vi "test2.vi"   [LabVIEW 2012]
uses:
  <vilib>/NXT/Dual Mode Library/Waits/Wait_Num.vi
types:
  T1 = typedef "LVHSConnector.ctl" = cluster{"Hardware":string, "Flattened String":string}
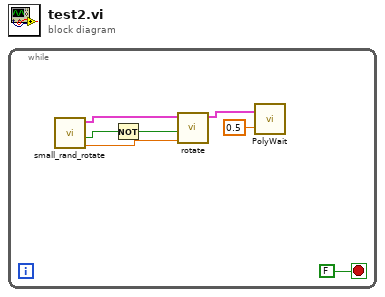
[diagram p0: block diagram]
diagram:
  n1 = while {
    stop <- FALSE stop-if-true
    n2 = call "small_rand_rotate.vi"() -> ("degrees rotated"=w6:dbl, "right(T)/left(F)"=w5:bool, "NXT"=w7:T1)  [unwired: 9 in]
    n3 = Not(x=w5) -> (.not. x?=w4:bool)
    n4 = call "rotate.vi"("degrees to  rotate"=w6, "right(T)/left(F)"=w4, "NXT 2"=w7) -> ("NXT"=w2:T1)  [unwired: 8 in]
    n5 = call-poly <vilib>:"PolyWait.vi"("Time (1 sec)"=sgl 0.5, "NXT"=w2) -> ()  [unwired: 2 in, 1 out]
  }
